vi "3_UpdateSubscribeList.vi"(8 "error in (no error)":errorcluster caption="错误输入（无错误）", 9 "T:Add":bool, 10 "Topic":string, 11 "MQTT_Client_Actor 输入":refnum<class "MQTT_Client_Actor.lvclass">) -> (0 "error out":errorcluster caption="错误输出", 3 "MQTT_Client_Actor 输出":refnum<class "MQTT_Client_Actor.lvclass">)   [LabVIEW 2018, in "MQTT_Client_Actor.lvlib" / "MQTT_Client_Actor.lvclass"]
uses:
  MQTT_Client_Actor.lvclass
  MQTT_Client_Actor.lvclass/MQTT_Client_Actor.ctl
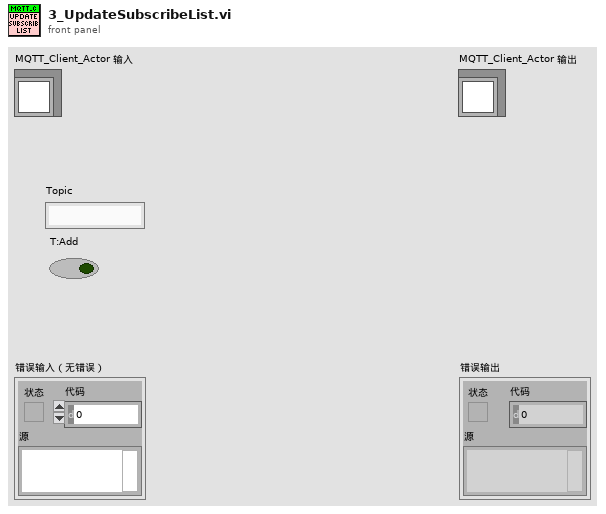
[diagram p1: front panel]
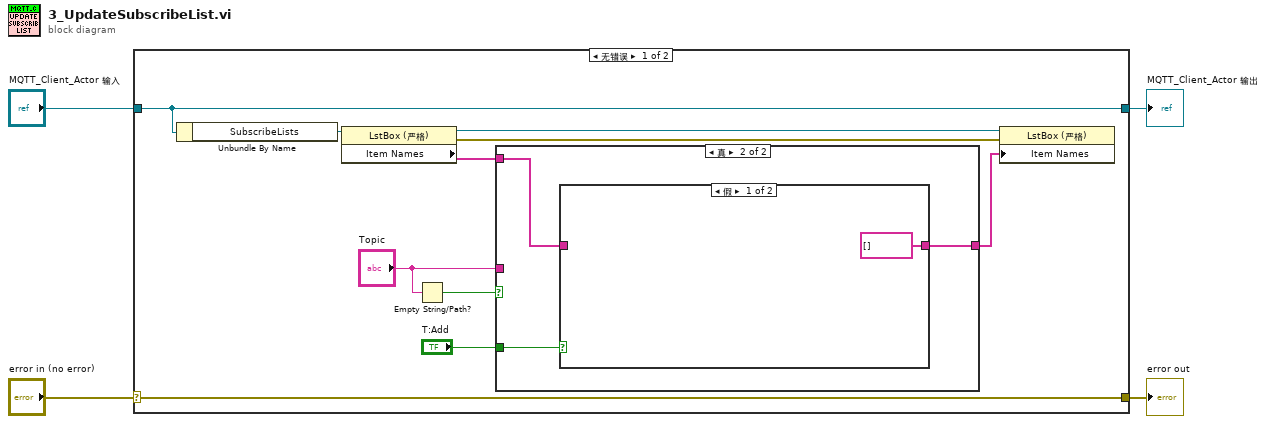
[diagram p0: block diagram]
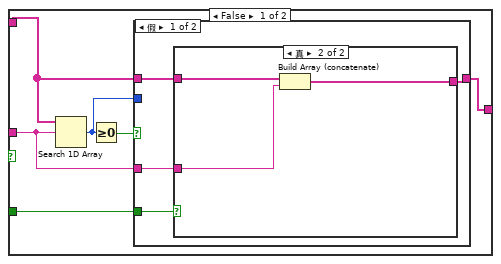
[diagram p2: hidden frame]
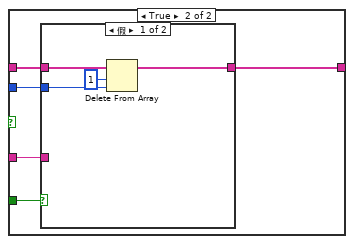
[diagram p4: hidden frame]
diagram:
  n1 = case shown="无错误" "error in (no error)" {
    selector: "error in (no error)" -> [w14 w45]
    tunnel: [w14 w45] -> w3
    tunnel: [w13 w44] -> w1
    tunnel: "MQTT_Client_Actor 输入" -> [w13 w44]
    frame No Error {
      n2 = Unbundle By Name(w13) -> ("SubscribeLists"=w12:refnum<vi>)
      n3 = property class="LstBox (严格)"(reference=w12) -> (reference out=w8:refnum<vi>, error out=w9:errorcluster, "Item Names"=w11:string[])  [unwired: 1 in]
      n4 = Empty String/Path?(string/path="Topic") -> (empty?=w6:bool)
      n5 = case shown="真" w6 {
        tunnel: w11 -> [w19 w39]
        tunnel: [w18 w40] -> w10
        tunnel: "Topic" -> [w16 _]
        tunnel: "T:Add" -> [w15 w41]
        frame False {
          n6 = Search 1D Array(1D array=w19, element=w16) -> (index of element=w17:i32)  [unwired: 1 in]
          n7 = Greater Or Equal To 0?(x=w17) -> (x >= 0?=w20:bool)
          n8 = case shown="假" w20 {
            tunnel: w19 -> [w24 w33]
            tunnel: [w23 w32] -> w18
            tunnel: w16 -> [w22 w31]
            tunnel: w15 -> [w21 w30]
            tunnel: w17 -> [_ w29]
            frame False {
              n9 = case shown="真" w21 {
                tunnel: w24 -> [w25 w28]
                tunnel: [w25 w27] -> w23
                tunnel: w22 -> [_ w26]
                frame False {
                }
                frame True {
                  n10 = Build Array (concatenate)(w28, w26) -> (w27:string[])
                }
              }
            }
            frame True {
              n11 = case shown="假" w30 {
                tunnel: w33 -> [w37 w38]
                tunnel: [w36 w38] -> w32
                tunnel: w31 -> [_ _]
                tunnel: w29 -> [w35 _]
                frame False {
                  n12 = Delete From Array(array=w37, length=1 ("长度"), index=w35) -> (array with subset deleted=w36:string[])  [unwired: 1 out]
                }
                frame True {
                }
              }
            }
          }
        }
        frame True {
          n13 = case shown="假" w41 {
            tunnel: [string[] [] ("Item Names") w43] -> w40
            tunnel: w39 -> [_ w43]
            frame False {
            }
            frame True {
            }
          }
        }
      }
      n14 = property class="LstBox (严格)"(reference=w8, error in=w9, "Item Names"=w10) -> ()  [unwired: 2 out]
    }
    frame Error {
    }
  }
  "error out" <- w3
  "MQTT_Client_Actor 输出" <- w1
